vi "toggle.vi"() -> ()   [LabVIEW 2015]
panel:
  in  "Auto?":bool=TRUE
  in  "timer":u32=250
  in  "stop":bool
  out "Boolean Output":bool
  in  "User Input":bool
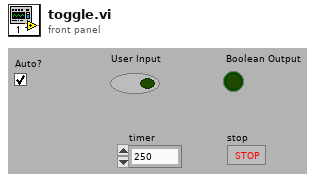
[diagram p1: front panel]
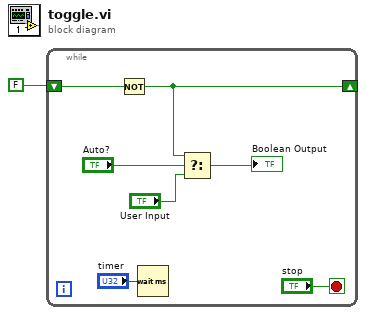
[diagram p0: block diagram]
diagram:
  n1 = while {
    shift-right: [w4] -> _
    shift-left: FALSE ("Boolean") -> [w8]
    stop <- "stop" stop-if-true
    n2 = Not(x=w8) -> (.not. x?=w4:bool)
    n3 = Wait (ms)(milliseconds to wait="timer") -> ()  [unwired: 1 out]
    n4 = Select(t=w4, s="Auto?", f="User Input") -> (s? t:f=→"Boolean Output":bool)
  }
